vi "Tango.vi"(9 "Stage Action":T1={"Action"=enum."Get Position", "Axis"=[], "Setpoint"=[], "Velocity"=0.5, "Cmd Recvd?"=FALSE, "Position"=[], "Status"=enum."Error", "Misc"=variant} {"Velocity" min=0.0 max=1.0 step=0.01}, 10 "Scan IM Notifier":refnum<notifier>, 11 "Tango Handle":i32) -> (3 "Tango Handle":i32)   [LabVIEW 2020]
uses:
  Stages Controls/Stage Notifier Element.ctl
  Stages Controls/Stage Actions.ctl
  Stages Controls/Stage Status.ctl
  <userlib>/Tango_DLL/Tango_DLL.lvlib
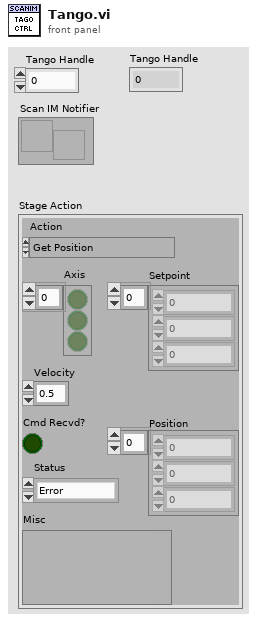
[diagram p1: front panel]
types:
  T1 = typedef "Stage Notifier Element.ctl" = cluster{"Action":T2, "Axis":bool[], "Setpoint":dbl[], "Velocity":dbl, "Cmd Recvd?":bool, "Position":dbl[], "Status":T3, "Misc":variant}
  T2 = typedef "Stage Actions.ctl" = enum16{"Get Position", "MVR", "MOVE", "HALT", "ONTARGET", "ERROR", "REFERENCE", "INIT", "VELOCITY", "STATUS", "EXIT", "HOME", "ZEROPOS", "NANOPOS", "ANALOG", "QUIT"}
  T3 = typedef "Stage Status.ctl" = enum16{"Error", "Abort", "Busy", "On Target"}
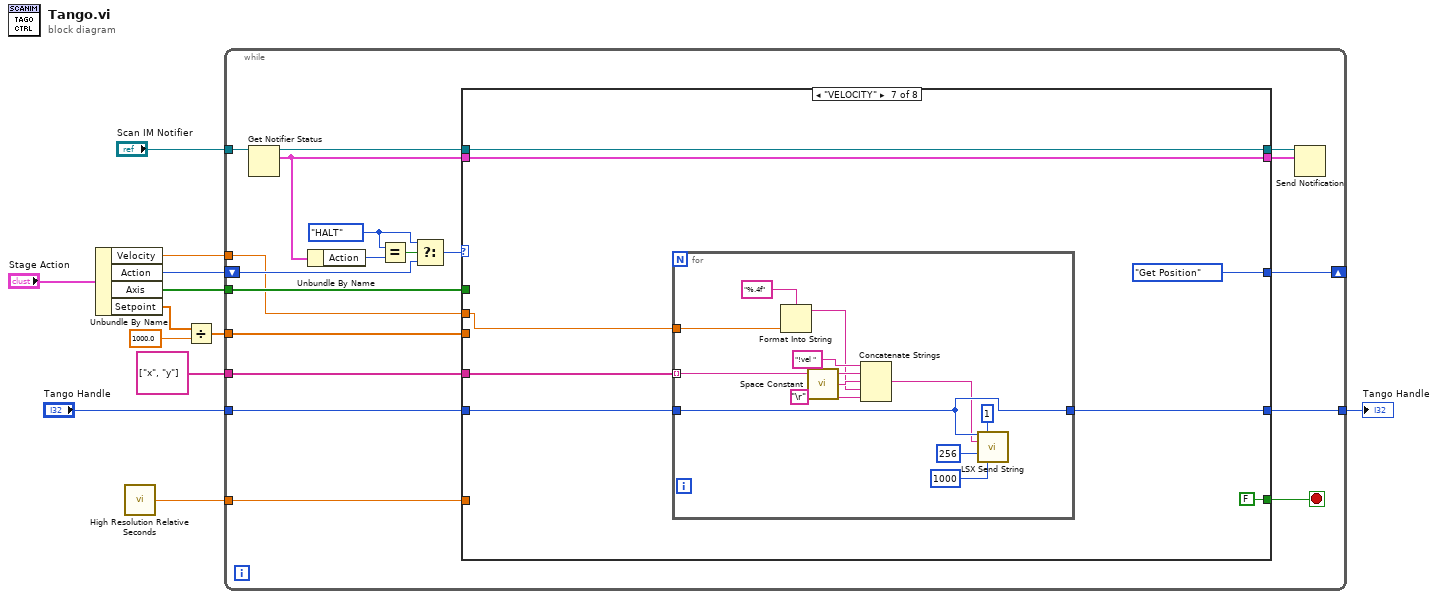
[diagram p0: block diagram]
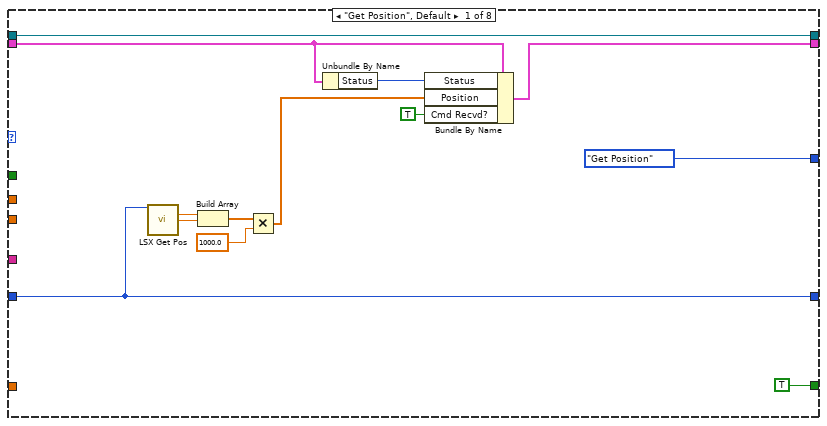
[diagram p2: hidden frame]
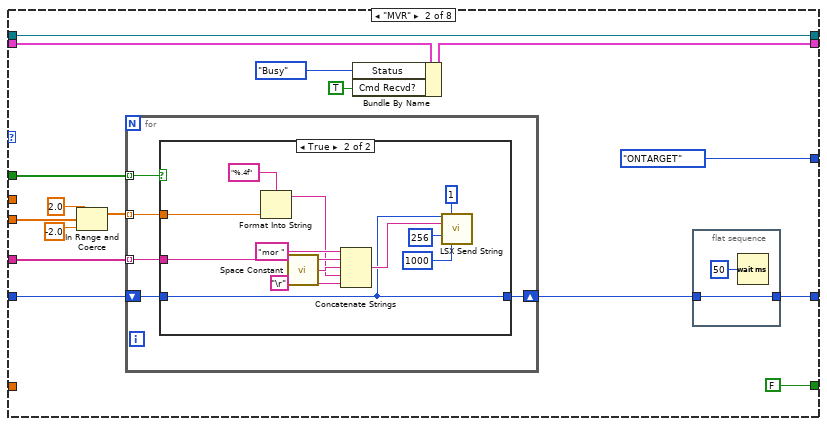
[diagram p3: hidden frame]
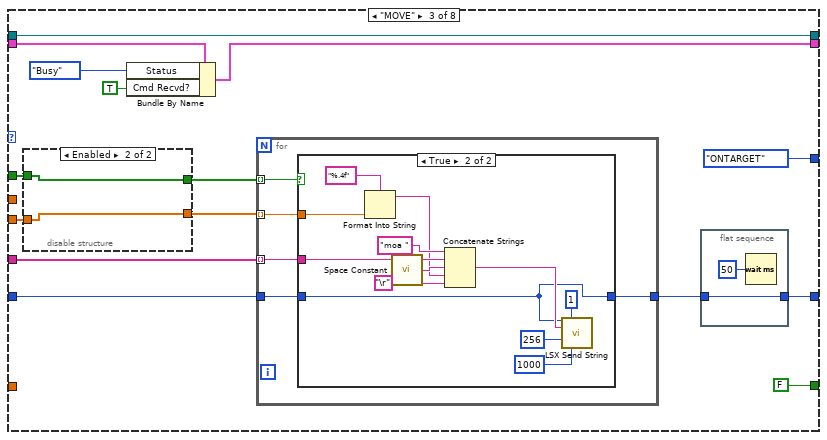
[diagram p5: hidden frame]
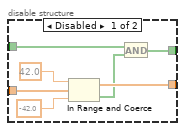
[diagram p6: hidden frame]
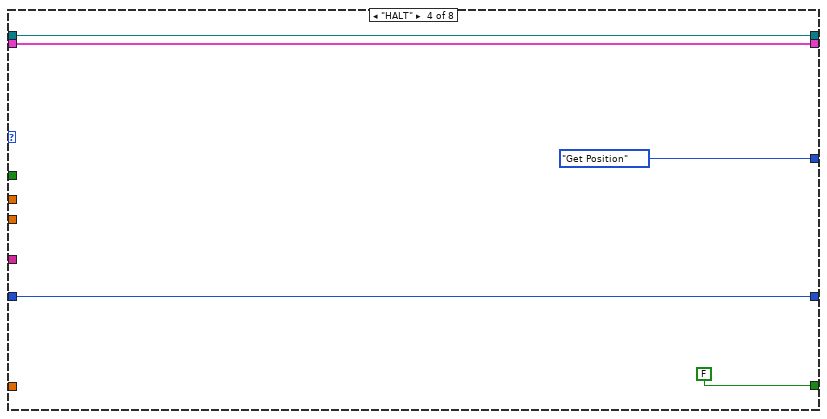
[diagram p8: hidden frame]
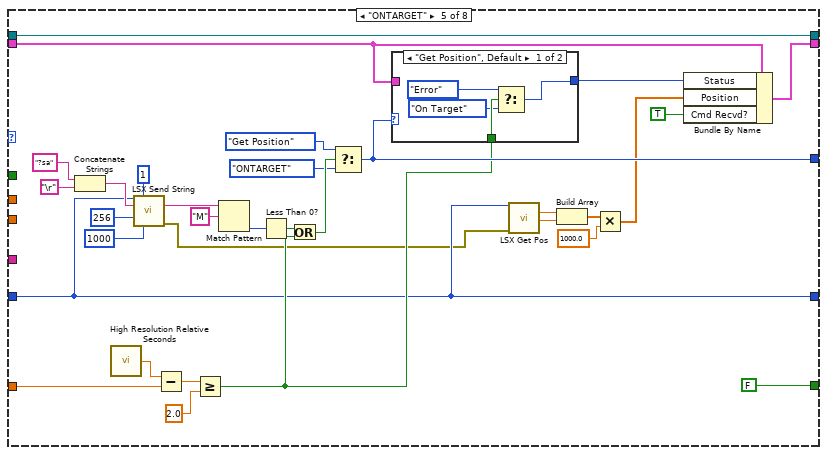
[diagram p9: hidden frame]
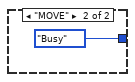
[diagram p10: hidden frame]
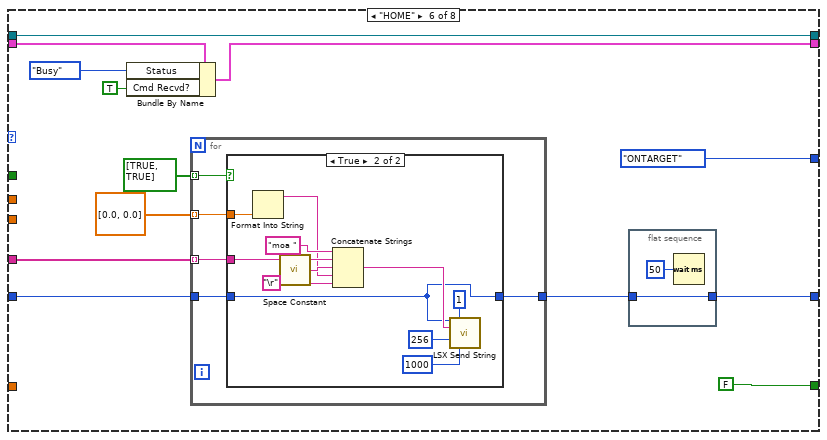
[diagram p11: hidden frame]
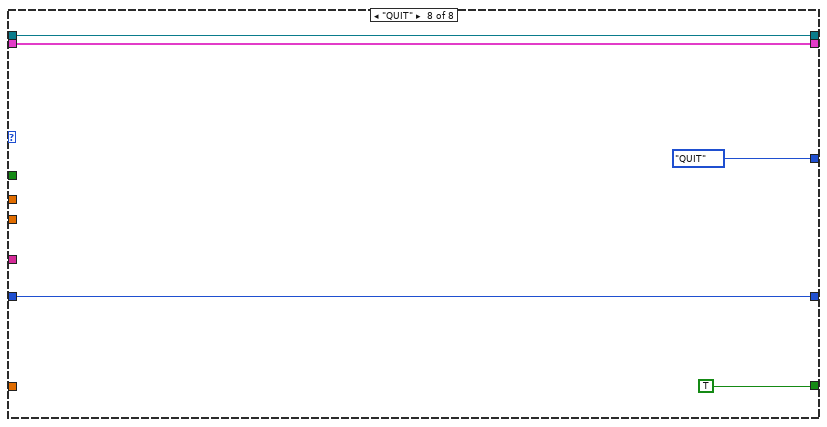
[diagram p13: hidden frame]
diagram:
  n1 = Unbundle By Name("Stage Action") -> ("Velocity"=w1:dbl, "Action"=w6:T2, "Axis"=w9:bool[], "Setpoint"=w4:dbl[])
  n2 = call <vilib>:"High Resolution Relative Seconds.vi"() -> ("relative seconds"=w8:dbl)
  n3 = Divide(x=w4, y=1000.0) -> (x/y=w2:dbl[])
  n4 = while {
    shift-right: [w29] -> _
    shift-left: w6 -> [w17]
    tunnel: "Tango Handle" -> [w30]
    tunnel: [w28] -> w12
    tunnel: w9 -> [w27]
    tunnel: "Scan IM Notifier" -> [w23]
    tunnel: w8 -> [w21]
    tunnel: w2 -> [w26]
    tunnel: string[] ["x", "y"] -> [w14]
    tunnel: w1 -> [w13]
    stop <- w31 stop-if-true
    w15 = Stage_Actions."HALT" ("x")
    n5 = Get Notifier Status(notifier=w23) -> (notifier out=w22:refnum<notifier>, current notification=w19:T1)  [unwired: 1 in, 3 out]
    n6 = Unbundle By Name(w19) -> ("Action"=w20:T2)
    n7 = Equal?(x=w15, y=w20) -> (x = y?=w18:bool)
    n8 = Select(t=w15, s=w18, f=w17) -> (s? t:f=w16:T2)
    n9 = case shown="\"VELOCITY\"" w16 {
      tunnel: [TRUE FALSE FALSE FALSE FALSE FALSE FALSE TRUE] -> w31
      tunnel: w30 -> [w34 w60 w95 w129 w134 w179 w202 w219]
      tunnel: [Stage_Actions."Get Position" ("x") Stage_Actions."ONTARGET" ("x") Stage_Actions."ONTARGET" ("x") Stage_Actions."Get Position" ("x") w157 Stage_Actions."ONTARGET" ("x") Stage_Actions."Get Position" ("x") Stage_Actions."QUIT" ("x")] -> w29
      tunnel: [w34 w54 w92 w129 w134 w178 w199 w219] -> w28
      tunnel: w27 -> [_ w59 w82 _ _ _ _ _]
      tunnel: w26 -> [_ w56 w94 _ _ _ _ _]
      tunnel: w22 -> [w41 w49 w87 w127 w156 w173 w205 w222]
      tunnel: [w41 w49 w87 w127 w156 w173 w205 w222] -> w25
      tunnel: [w42 w50 w88 w126 w160 w174 w204 w221] -> w24
      tunnel: w19 -> [w40 w48 w86 w126 w158 w172 w204 w221]
      tunnel: w21 -> [_ _ _ _ w159 _ _ _]
      tunnel: w14 -> [_ w45 w83 _ _ w169 w201 _]
      tunnel: w13 -> [_ _ _ _ _ _ w200 _]
      frame "Get Position", Default {
        n10 = call <userlib>:"LSX Get Pos.vi"("lLSID"=w34) -> ("pdX out"=w36:dbl, "pdY out"=w35:dbl)  [unwired: 9 in, 4 out]
        n11 = Build Array(w36, w35) -> (w38:dbl[])
        n12 = Multiply(x=w38, y=1000.0) -> (x*y=w33:dbl[])
        n13 = Unbundle By Name(w40) -> ("Status"=w39:T3)
        n14 = Bundle By Name(cluster=w40, "Status"=w39, "Position"=w33, "Cmd Recvd?"=TRUE) -> (w42:T1)
      }
      frame "MVR" {
        n15 = In Range and Coerce(upper limit=2.0, x=w56, lower limit=-2.0) -> (coerced(x)=w55:dbl[])  [unwired: 1 out]
        n16 = for {
          shift-right: [w66] -> w53
          shift-left: w60 -> [w67]
          tunnel: w59 -> [w65] mode=indexing
          tunnel: w55 -> [w64] mode=indexing
          tunnel: w45 -> [w63] mode=indexing
          n17 = case shown="True" w65 {
            tunnel: w67 -> [w68 w70]
            tunnel: [w68 w70] -> w66
            tunnel: w64 -> [_ w78]
            tunnel: w63 -> [_ w76]
            frame False {
            }
            frame True {
              n18 = Format Into String(format string="%.4f", w78) -> (resulting string=w74:string)  [unwired: 2 in, 1 out]
              n19 = call <vilib>:"Space Constant.vi"() -> ("String"=w75:string)
              n20 = Concatenate Strings("mor ", w76, w75, w74, "\r") -> (w73:string)
              n21 = call <userlib>:"LSX Send String.vi"("lLSID"=w70, "bReadLine"=1, "pcStr"=w73, "lMaxLen"=256, "lTimeOut"=1000) -> ()  [unwired: 7 in, 4 out]
            }
          }
        }
        n22 = Bundle By Name(cluster=w48, "Status"=Stage_Status."Busy", "Cmd Recvd?"=TRUE) -> (w50:T1)
        n23 = flat-sequence {
          tunnel: [w62] -> w54
          tunnel: w53 -> [w62]
          frame #0 {
            n24 = Wait (ms)(milliseconds to wait=u32 50) -> ()  [unwired: 1 out]
          }
        }
      }
      frame "MOVE" {
        n25 = disable-structure shown="Enabled" {
          disable-tunnel: w94 -> [w100 w103]
          disable-tunnel: [w99 w103] -> w93
          disable-tunnel: w82 -> [w97 w104]
          disable-tunnel: [w96 w104] -> w81
          frame Disabled {
            n26 = In Range and Coerce(upper limit=42.0, x=w100, lower limit=-42.0) -> (coerced(x)=w99:dbl[], In Range?=w98:bool[])
            n27 = And(x=w97, y=w98) -> (x .and. y?=w96:bool[])
          }
          frame Enabled {
          }
        }
        n28 = Bundle By Name(cluster=w86, "Status"=Stage_Status."Busy", "Cmd Recvd?"=TRUE) -> (w88:T1)
        n29 = for {
          tunnel: w81 -> [w109] mode=indexing
          tunnel: w93 -> [w108] mode=indexing
          tunnel: w83 -> [w107] mode=indexing
          tunnel: w95 -> [w111]
          tunnel: [w110] -> w91
          n30 = case shown="True" w109 {
            tunnel: w111 -> [w112 w114]
            tunnel: [w112 w114] -> w110
            tunnel: w108 -> [_ w122]
            tunnel: w107 -> [_ w120]
            frame False {
            }
            frame True {
              n31 = Format Into String(format string="%.4f", w122) -> (resulting string=w118:string)  [unwired: 2 in, 1 out]
              n32 = call <vilib>:"Space Constant.vi"() -> ("String"=w119:string)
              n33 = Concatenate Strings("moa ", w120, w119, w118, "\r") -> (w117:string)
              n34 = call <userlib>:"LSX Send String.vi"("lLSID"=w114, "bReadLine"=1, "pcStr"=w117, "lMaxLen"=256, "lTimeOut"=1000) -> ()  [unwired: 7 in, 4 out]
            }
          }
        }
        n35 = flat-sequence {
          tunnel: [w106] -> w92
          tunnel: w91 -> [w106]
          frame #0 {
            n36 = Wait (ms)(milliseconds to wait=u32 50) -> ()  [unwired: 1 out]
          }
        }
      }
      frame "HALT" {
      }
      frame "ONTARGET" {
        n37 = Concatenate Strings("?sa" ("pcStr"), "\r") -> (w141:string)
        n38 = call <vilib>:"High Resolution Relative Seconds.vi"() -> ("relative seconds"=w153:dbl)
        n39 = call <userlib>:"LSX Send String.vi"("lLSID"=w134, "bReadLine"=1, "pcStr"=w141, "lMaxLen"=256, "lTimeOut"=1000) -> ("pcStr out"=w140:string, "error out"=w131:errorcluster)  [unwired: 7 in, 2 out]
        n40 = Subtract(x=w153, y=w159) -> (x-y=w152:dbl)
        n41 = Greater Or Equal?(x=w152, y=2.0) -> (x >= y?=w150:bool)
        n42 = Match Pattern(string=w140, regular expression="M") -> (offset past match=w138:i32)  [unwired: 1 in, 3 out]
        n43 = Less Than 0?(x=w138) -> (x < 0?=w137:bool)
        n44 = Or(x=w137, y=w150) -> (x .or. y?=w155:bool)
        n45 = Select(t=Stage_Actions."Get Position" ("x"), s=w155, f=Stage_Actions."ONTARGET" ("x")) -> (s? t:f=w157:T2)
        n46 = case shown="\"Get Position\", Default" w157 {
          tunnel: w158 -> [_ _]
          tunnel: [w164 Stage_Status."Busy" ("Status")] -> w147
          tunnel: w150 -> [w165 _]
          frame "Get Position", Default {
            n47 = Select(t=Stage_Status."Error" ("Status"), s=w165, f=Stage_Status."On Target" ("Status")) -> (s? t:f=w164:T3)
          }
          frame "MOVE" {
          }
        }
        n48 = call <userlib>:"LSX Get Pos.vi"("lLSID"=w134, "error in (no error)"=w131) -> ("pdX out"=w136:dbl, "pdY out"=w135:dbl)  [unwired: 8 in, 4 out]
        n49 = Build Array(w136, w135) -> (w133:dbl[])
        n50 = Multiply(x=w133, y=1000.0) -> (x*y=w130:dbl[])
        n51 = Bundle By Name(cluster=w158, "Status"=w147, "Position"=w130, "Cmd Recvd?"=TRUE) -> (w160:T1)
      }
      frame "HOME" {
        n52 = Bundle By Name(cluster=w172, "Status"=Stage_Status."Busy", "Cmd Recvd?"=TRUE) -> (w174:T1)
        n53 = for {
          tunnel: bool[] [TRUE, TRUE] -> [w184] mode=indexing
          tunnel: dbl[] [0.0, 0.0] -> [w183] mode=indexing
          tunnel: w169 -> [w182] mode=indexing
          tunnel: w179 -> [w186]
          tunnel: [w185] -> w177
          n54 = case shown="True" w184 {
            tunnel: w186 -> [w187 w188]
            tunnel: [w187 w188] -> w185
            tunnel: w183 -> [_ w196]
            tunnel: w182 -> [_ w194]
            frame False {
            }
            frame True {
              n55 = Format Into String(w196) -> (resulting string=w192:string)  [unwired: 3 in, 1 out]
              n56 = call <vilib>:"Space Constant.vi"() -> ("String"=w193:string)
              n57 = Concatenate Strings("moa ", w194, w193, w192, "\r") -> (w191:string)
              n58 = call <userlib>:"LSX Send String.vi"("lLSID"=w188, "bReadLine"=1, "pcStr"=w191, "lMaxLen"=256, "lTimeOut"=1000) -> ()  [unwired: 7 in, 4 out]
            }
          }
        }
        n59 = flat-sequence {
          tunnel: [w181] -> w178
          tunnel: w177 -> [w181]
          frame #0 {
            n60 = Wait (ms)(milliseconds to wait=u32 50) -> ()  [unwired: 1 out]
          }
        }
      }
      frame "VELOCITY" {
        n61 = for {
          tunnel: w200 -> [w217]
          tunnel: w201 -> [w216] mode=indexing
          tunnel: w202 -> [w218]
          tunnel: [w218] -> w199
          n62 = Format Into String(format string="%.4f", w217) -> (resulting string=w211:string)  [unwired: 2 in, 1 out]
          n63 = call <vilib>:"Space Constant.vi"() -> ("String"=w212:string)
          n64 = Concatenate Strings("!vel ", w216, w212, w211, "\r") -> (w210:string)
          n65 = call <userlib>:"LSX Send String.vi"("lLSID"=w218, "bReadLine"=1, "pcStr"=w210, "lMaxLen"=256, "lTimeOut"=1000) -> ()  [unwired: 7 in, 4 out]
        }
      }
      frame "QUIT" {
      }
    }
    n66 = Send Notification(notification=w24, notifier=w25) -> ()  [unwired: 1 in, 2 out]
  }
  "Tango Handle" <- w12
